vi "backup.vi"() -> ()   [LabVIEW 2017]
uses:
  <vilib>/myRIO/Instrument Drivers/Utilities/Utilities.lvlib
  qsm/type defs/states.ctl
  qsm/type defs/task.ctl
  qsm/type defs/action buttons.ctl
panel:
  in  "ctl num":i32
  out "ball match":bool
  in  "?":i32
  in  "?":i32
  in  "?":i32
  in  "?":i32
  in  "?":i32
  in  "action buttons":T1
  out "y0 (circle)":i32
  out "x0 (circle)":i32
  out "x1 (circle)":i32
  out "y1 (circle)":i32
  in  "divider (circle)":sgl=1.0
  out "Radius (circle)":dbl
  out "Circles Calibrated (Shape Detection 1)":T2(array[cluster]) {"Position"."Y" format="%.2f"; "Position"."X" format="%.2f"}
  in  "ROI Descriptor COLOR Mask":T3={"Global Rectangle"=[0, 0, 0, 0], "Contours"=[{"ID"=enum."External", "Type"=0, "Coordinates"=[0, 0, 0, 0]}]}
  in  "ROI Descriptor (COLOR Mask 1)":T3={"Global Rectangle"=[51, 157, 345, 350], "Contours"=[{"ID"=enum."External", "Type"=5, "Coordinates"=[137, 230, 93, 226, 75, 199, 49, 200, 56, 145, 98, 111, 200, 119, 250, 126, 235, 166, 240, 212, 188, 243, 303, 244, 336, 247, 336, 271, 335, 292, 335, 318, 314, 323, 293, 334, 279, 345, 272, 349, 187, 349, 186, 335, 120, 334, 112, 314, 100, 297, 59, 291, 51, 288, 51, 287]}]} {"Contours"."Type" items=["No Selection", "Point", "Line", "Rectangle", "Oval", "Polygon", "Freehand Region", "Annulus", "Unused2", "Unused3", "Broken Line", "Freehand Line", "Rotated Rectangle"]}
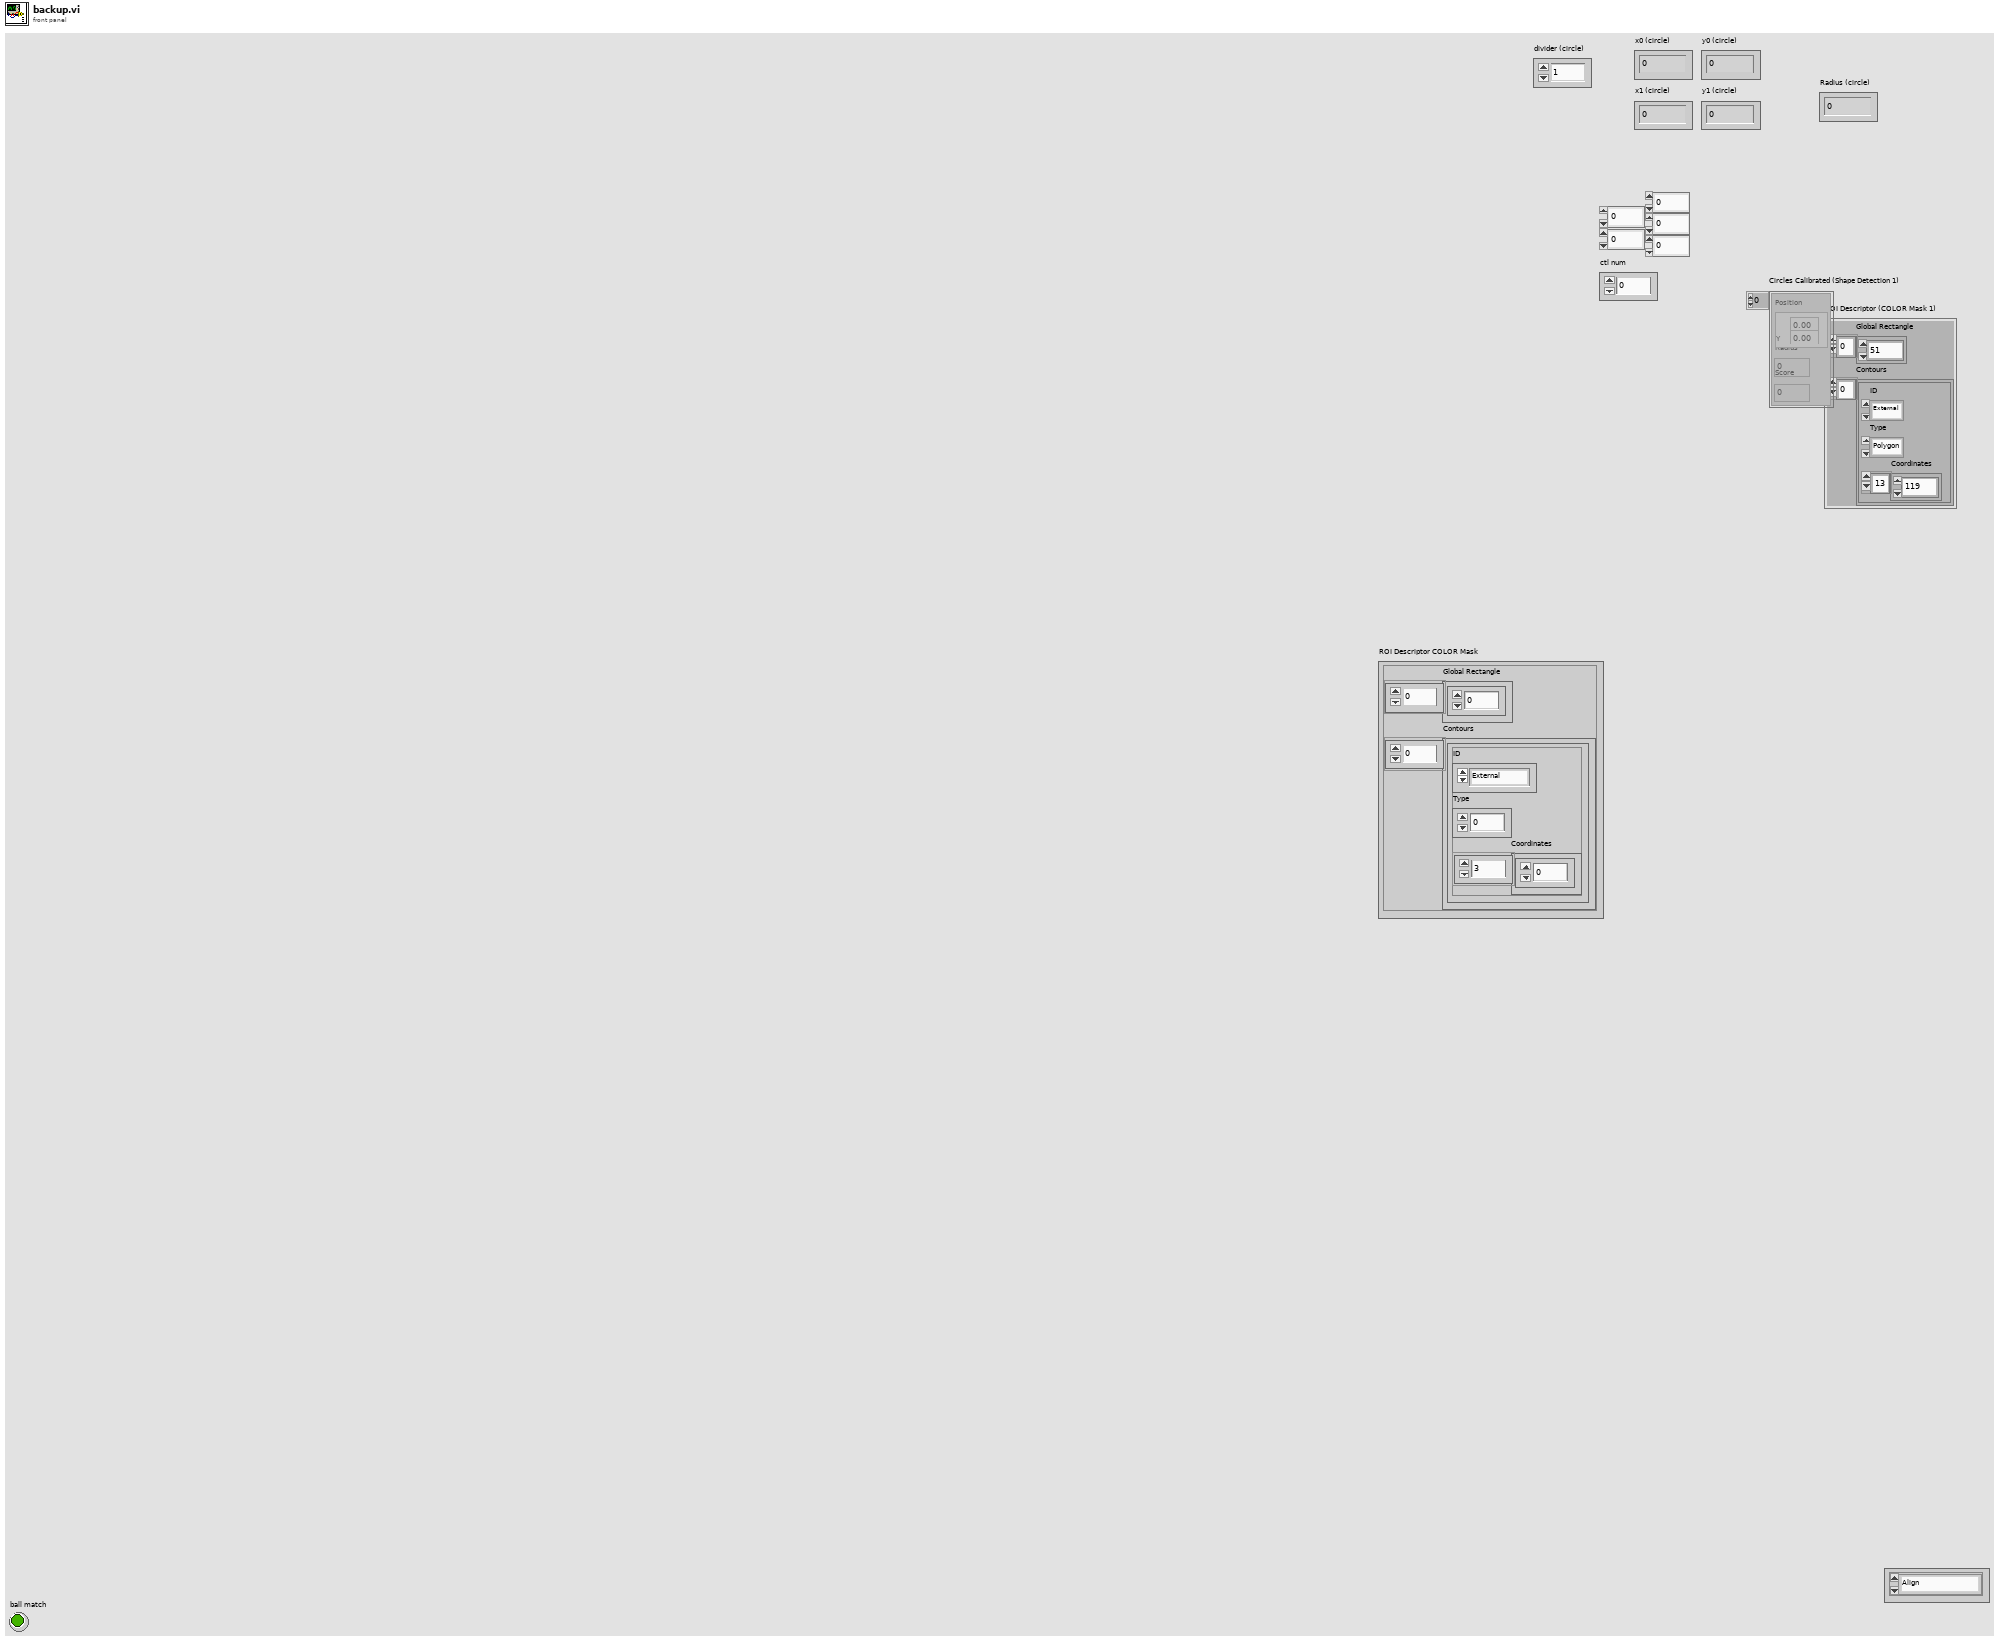
[diagram p1: front panel]
types:
  T1 = typedef "action buttons.ctl" = cluster{"Shape - t, Color - f":enum16{"Align", "(pattern) Align", "Pattern", "(mod) pattern", "<mod>[P] remembering", "<mod>[P] go through tunnel", "<mod>[P] comparing", "(mod) ball", "Ball", "Other", "Clear", "navx", "Joystick control"}}
  T2 = cluster{"Position":cluster{"X":sgl, "Y":sgl}, "Radius":dbl, "Score":dbl}[]
  T3 = cluster{"Global Rectangle":i32[], "Contours":cluster{"ID":enum32{"External", "Internal"}, "Type":u32, "Coordinates":i32[]}[]}
  T4 = enum16{"Align", "(pattern) Align", "Pattern", "(mod) pattern", "(mod) ball", "Ball", "Other", "Clear", "Joystick control"}
  T5 = enum16{"Align", "(pattern) Align", "Pattern", "(mod) pattern", "Ball", "Other", "Clear", "Joystick control"}
  T6 = typedef "task.ctl" = T7[]
  T7 = typedef "states.ctl" = enum16{"(qsm) schedule", "(qsm) initialize", "(qsm) release", "(qsm) clean up", "(qsm) shutdown", "(myRIO) initialize", "(myRIO) clean up", "(myRIO) update ports", "Setup get", "(image) get", "(image) show", "(ball) Shape detection", "(ball) Calc ball indx", "(ball) Calculate ROI", "(ball) Analyze color", "(ball) Align", "(ball) Wait", "(ball) Grab", "(pattern) Find Square", "(pattern) Calculate ROI", "(pattern) Calc pattern indx", "(pattern) Compare", "(pattern) Analyze pattern", "(pattern) Align", "(pattern) Wait", "(joystick) Joystick control", "_Timer", "Wait for button"}
  T8 = typedef "states.ctl" = enum16{"(qsm) schedule", "(qsm) initialize", "(qsm) release", "(qsm) clean up", "(qsm) shutdown", "(myRIO) initialize", "(myRIO) clean up", "(myRIO) update ports", "Setup get", "(image) get", "(image) show", "(ball) Shape detection", "(ball) Calc ball indx", "(ball) Calculate ROI", "(ball) Analyze color", "(ball) Align", "(ball) Wait", "(ball) Grab", "(pattern) Find Square", "(pattern) Calculate ROI", "(pattern) Calc pattern indx", "Compare", "(pattern) Analyze pattern", "(pattern) Align", "(pattern) Wait", "(pattern) states control", "navx", "(joystick) Joystick control", "_Timer", "Wait for button"}
  T9 = cluster{"Position":cluster{"X":sgl, "Y":sgl}, "Radius":dbl, "Score":dbl}
  T10 = cluster{"ID":enum32{"External", "Internal"}, "Type":u32, "Coordinates":i32[]}[]
  T11 = cluster{"ID":enum32{"External", "Internal"}, "Type":u32, "Coordinates":i32[]}
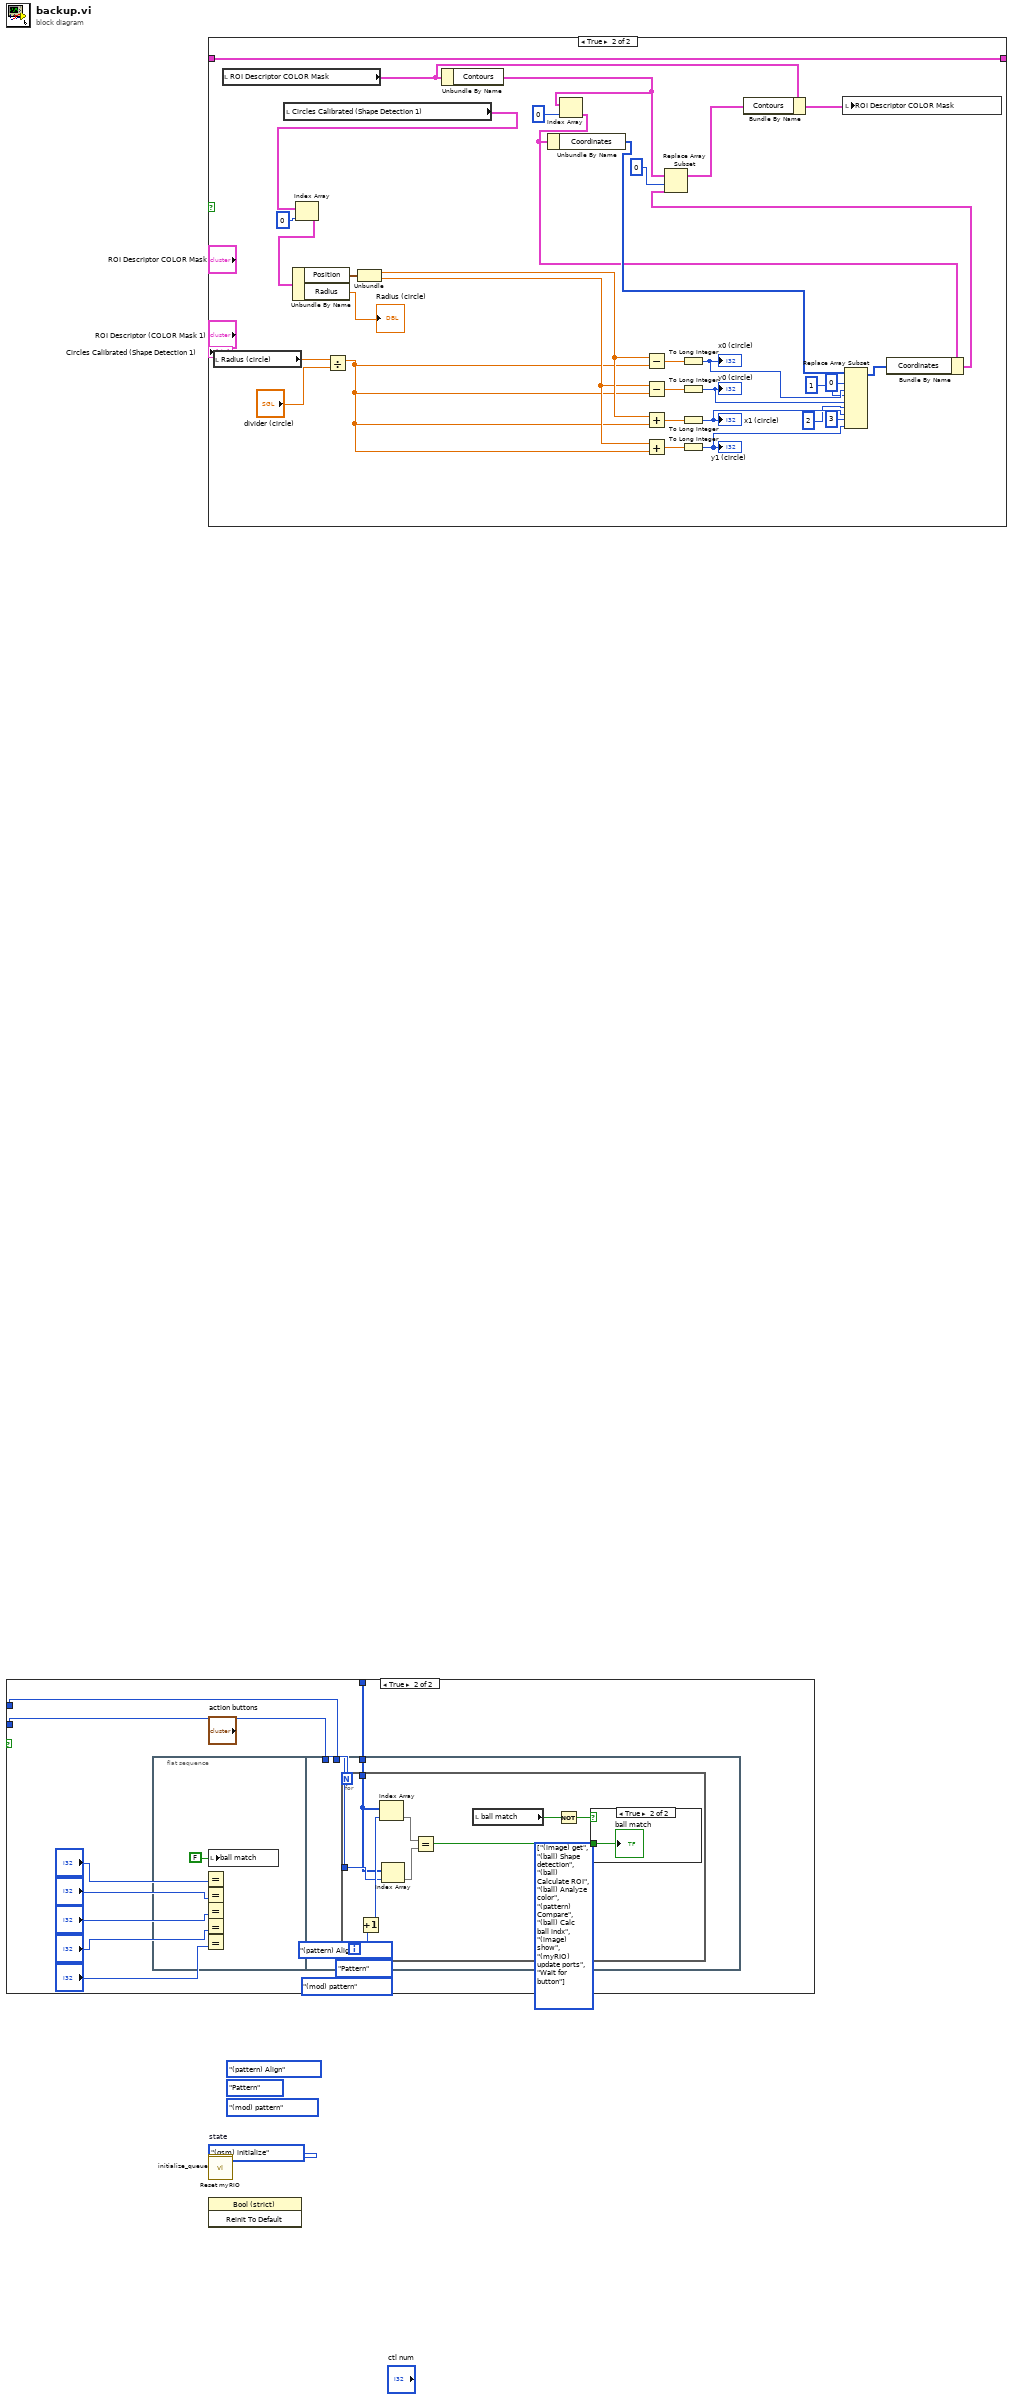
[diagram p0: block diagram]
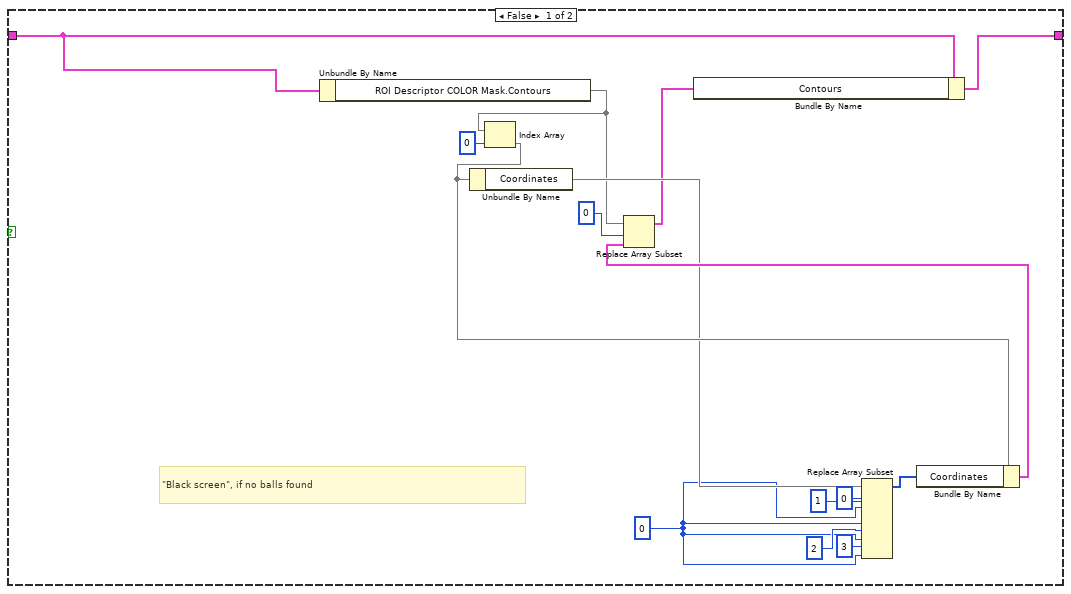
[diagram p4: hidden frame]
diagram:
  (unwired) T4."(mod) pattern" ("Shape - t, Color - f")
  (unwired) T4."Pattern" ("Shape - t, Color - f")
  (unwired) T4."(pattern) Align" ("Shape - t, Color - f")
  (unwired) T5."(mod) pattern" ("y")
  (unwired) T5."Pattern" ("y")
  (unwired) T5."(pattern) Align" ("y")
  (unwired) T6 [enum."(image) get", enum."(ball) Shape detection", enum."(ball) Calculate ROI", enum."(ball) Analyze color", enum."(pattern) Compare", enum."(ball) Calc ball indx", enum."(image) show", enum."(myRIO) update ports", enum."Wait for button"] items=["(qsm) schedule", "(qsm) initialize", "(qsm) release", "(qsm) clean up", "(qsm) shutdown", "(myRIO) initialize", "(myRIO) clean up", "(myRIO) update ports", "Setup get", "(image) get", "(image) show", "(ball) Shape detection", "(ball) Calc ball indx", "(ball) Calculate ROI", "(ball) Analyze color", "(ball) Align", "(ball) Wait", "(ball) Grab", "(pattern) Find Square", "(pattern) Calculate ROI", "(pattern) Calc pattern indx", "(pattern) Compare", "(pattern) Analyze pattern", "(pattern) Align", "(pattern) Wait", "(joystick) Joystick control", "_Timer", "Wait for button"] ("task")
  w6 = states."(qsm) initialize"  # state
  n1 = case shown="True" {
    selector: _ -> [_ _]
    tunnel: _ -> [_ w13]
    tunnel: _ -> [_ w12]
    tunnel: _ -> [_ w11]
    frame False {
    }
    frame True {
      n2 = flat-sequence {
        tunnel: w13 -> [w17]
        tunnel: w12 -> [w16]
        tunnel: w11 -> [w15]
        frame #0 {
          n3 = local write "ball match"(FALSE ("ball match")) -> ()
        }
        frame #1 {
          n4 = for {
            N: w17 -> [_]
            tunnel: w16 -> [w20]
            tunnel: w15 -> [w18]
            i -> [w22]
            n5 = Increment(x=w22) -> (x+1=w21:i32)
            n6 = Index Array(array=w18, index=w21) -> (element=w24)
            n7 = Index Array(array=w18, index=w20) -> (element=w23)
            n8 = Equal?(x=w24, y=w23) -> (x = y?=w25:bool)
            n9 = local read "ball match"() -> (w19:bool)
            n10 = Not(x=w19) -> (.not. x?=w26:bool)
            n11 = case shown="True" w26 {
              tunnel: w25 -> [_ w27]
              frame False {
              }
              frame True {
                "ball match" <- w27
              }
            }
          }
        }
      }
    }
  }
  n12 = Equal?(y="?") -> ()  [unwired: 1 in, 1 out]
  n13 = Equal?(y="?") -> ()  [unwired: 1 in, 1 out]
  n14 = Equal?(y="?") -> ()  [unwired: 1 in, 1 out]
  n15 = Equal?(y="?") -> ()  [unwired: 1 in, 1 out]
  n16 = Equal?(y="?") -> ()  [unwired: 1 in, 1 out]
  n17 = case shown="True" {
    selector: _ -> [_ _]
    tunnel: [w29 w43] -> _
    tunnel: _ -> [w28 w43]
    frame False {
      w30 = 0 ("index")
      # "\"Black screen\", if no balls found"
      n18 = Unbundle By Name(w28) -> ("ROI Descriptor COLOR Mask.Contours"=w37)
      n19 = Index Array(array=w37, index=0) -> (element=w40)
      n20 = Unbundle By Name(w40) -> ("Coordinates"=w39)
      n21 = Replace Array Subset(array=w39, new element #1=w30, index #1=0 ("index"), new element #2=w30, index #2=1 ("index"), new element #3=w30, index #3=2 ("index"), new element #4=w30, index #4=3 ("index")) -> (w41:i32[])
      n22 = Bundle By Name(cluster=w40, "Coordinates"=w41) -> (w42:cluster{})
      n23 = Replace Array Subset(array=w37, new element=w42, index=0) -> (w38:cluster{}[])
      n24 = Bundle By Name(cluster=w28, "Contours"=w38) -> (w29:cluster{})
    }
    frame True {
      n25 = local read "Radius (circle)"() -> (w50:dbl)
      n26 = local read "ROI Descriptor COLOR Mask"() -> (w45:T3)
      n27 = local read "Circles Calibrated (Shape Detection 1)"() -> (w75:T2)
      n28 = Index Array(array=w75, index=0) -> (element=w73:T9)
      n29 = Unbundle By Name(w73) -> ("Position"=w72:cluster{"X":sgl, "Y":sgl}, "Radius"=→"Radius (circle)":dbl)
      n30 = Divide(x=w50, y="divider (circle)") -> (x/y=w49:dbl)
      n31 = Unbundle(w72) -> ("X"=w69:sgl, "Y"=w68:sgl)
      n32 = Unbundle By Name(w45) -> ("Contours"=w47:T10)
      n33 = Index Array(array=w47, index=0) -> (element=w61:T11)
      n34 = Unbundle By Name(w61) -> ("Coordinates"=w63:i32[])
      n35 = Subtract(x=w69, y=w49) -> (x-y=w67:dbl)
      n36 = Subtract(x=w68, y=w49) -> (x-y=w66:dbl)
      n37 = Add(x=w69, y=w49) -> (x+y=w64:dbl)
      n38 = Add(x=w68, y=w49) -> (x+y=w65:dbl)
      n39 = To Long Integer(number=w67) -> (32bit integer=w58:i32)
      "x0 (circle)" <- w58
      n40 = To Long Integer(number=w66) -> (32bit integer=w57:i32)
      "y0 (circle)" <- w57
      n41 = To Long Integer(number=w64) -> (32bit integer=w56:i32)
      "x1 (circle)" <- w56
      n42 = To Long Integer(number=w65) -> (32bit integer=w55:i32)
      "y1 (circle)" <- w55
      n43 = Replace Array Subset(array=w63, new element #1=w58, index #1=0 ("index"), new element #2=w57, index #2=1 ("index"), new element #3=w56, index #3=2 ("index"), new element #4=w55, index #4=3 ("index")) -> (w60:i32[])
      n44 = Bundle By Name(cluster=w61, "Coordinates"=w60) -> (w59:T11)
      n45 = Replace Array Subset(array=w47, new element=w59, index=0) -> (w44:T10)
      n46 = Bundle By Name(cluster=w45, "Contours"=w44) -> (w46:T3)
      n47 = local write "ROI Descriptor COLOR Mask"(w46) -> ()
    }
  }
  n48 = call "initialize_queue.vi"("state"=w6) -> ("error out"=w7:errorcluster, "queue out"=w8:refnum<queue>)  [unwired: 9 in]
  n49 = call <vilib>:"Reset myRIO.vi"() -> ("error in (no error)"=w10:errorcluster)  [unwired: 10 in, 1 out]
  n50 = invoke on="Invoke Node" class="Bool (strict)" method="Reinit To Default"() -> ()  [unwired: 3 in, 3 out]
